vi "MyQH Main.vi"() -> ()   [LabVIEW 2014]
doc: "Diese Vorlage beschreibt das Design \"Handler für Nachrichten-Queues\".\n\nDie Schleife zur Ereignisbehandlung erzeugt Nachrichten basierend auf Benutzereingaben.\n\nDie Schleife zur Nachrichtenbehandlung verarbeitet Nachrichten, die von der Ereignisschleife oder anderen Nachrichten erzeugt wurden. Die Nachrichten sind String-Werte. Neue Nachrichten können also einfach der Case-Struktur der Nachrichtenschleife hinzugefügt werden. Der Nachrichten-Cluster kann auch einen optionalen Wert für Nachrichtendaten enthalten. Dabei handelt es sich um einen Variant, der in beliebige nachrichtenspezifische Daten umgewandelt werden kann."
uses:
  controls/ProtocolT.ctl
  controls/ProtocolEntry.ctl
  controls/MyQH UI Data.ctl
  support/Message Queue/Enqueue Message (Single).vi
  support/Message Queue/Enqueue Message (Array).vi
  <vilib>/Utility/error.llb/Error Cluster From Error Code.vi
  <vilib>/ErrorRing/Error Ring.xnode
  support/Message Queue/MyQH Message Queue.lvlib
  support/User Event - Stop/MyQH User Event - Stop.lvlib
panel:
  in  "ProtocolT":T1 {"Zeitstempel" format=" %<%X %x>T"}
  out "Anzeige <Ersetzen>":string
  in  "Remove Entry":bool
  in  "Add Entry":bool
  in  "Beenden":bool
  # "Für diese Elemente wurden Wertänderungs-Ereignisse in der Ereignisstruktur im Blockdiagramm konfiguriert.\n\nErsetzen Sie die Elemente durch für Ihre Anwendung gewünschte Elemente (und konfigurieren Sie die Ereignisstruktur neu)."
  # "Diese Vorlage beschreibt das Design für einen Handler für Nachrichten-Queues.\n\nWechseln Sie für weitere Informationen zum Blockdiagramm."
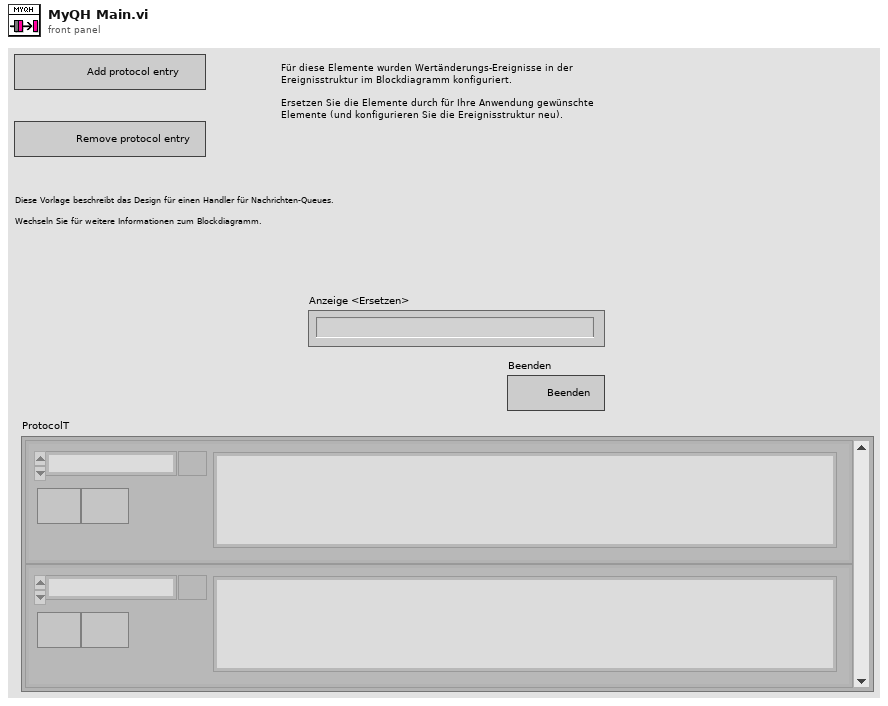
[diagram p1: front panel]
types:
  T1 = typedef "ProtocolT.ctl" = T2[]
  T2 = typedef "ProtocolEntry.ctl" = cluster{"Zeitstempel":timestamp, "String":string, "Abbrechen-Schaltfläche":bool, "Optionen-Schaltfläche":bool}
  T3 = typedef "MyQH UI Data.ctl" = cluster{"Boolesch <Ersetzen>":bool, "String <Ersetzen>":string, "Numerisch <Ersetzen>":dbl, "Etwas tun (Ref.)":refnum<vi>, "Etwas anderes tun (Ref.)":refnum<vi>, "Datenanzeige (Ref.)":refnum<vi>, "Beenden-Schaltfl. (Ref.)":refnum<vi>, "Cluster":cluster{"VI Referenz":refnum<vi>}, "Arr Referenz":refnum<vi>, "Cluster Referenz":refnum<vi>}
  T4 = cluster{"Status":bool, "Code":i32, "Quelle":string}
  T5 = typedef "MyQH Message Queue.lvlib/All Message Queues.ctl" = cluster{"UI":refnum<queue>}
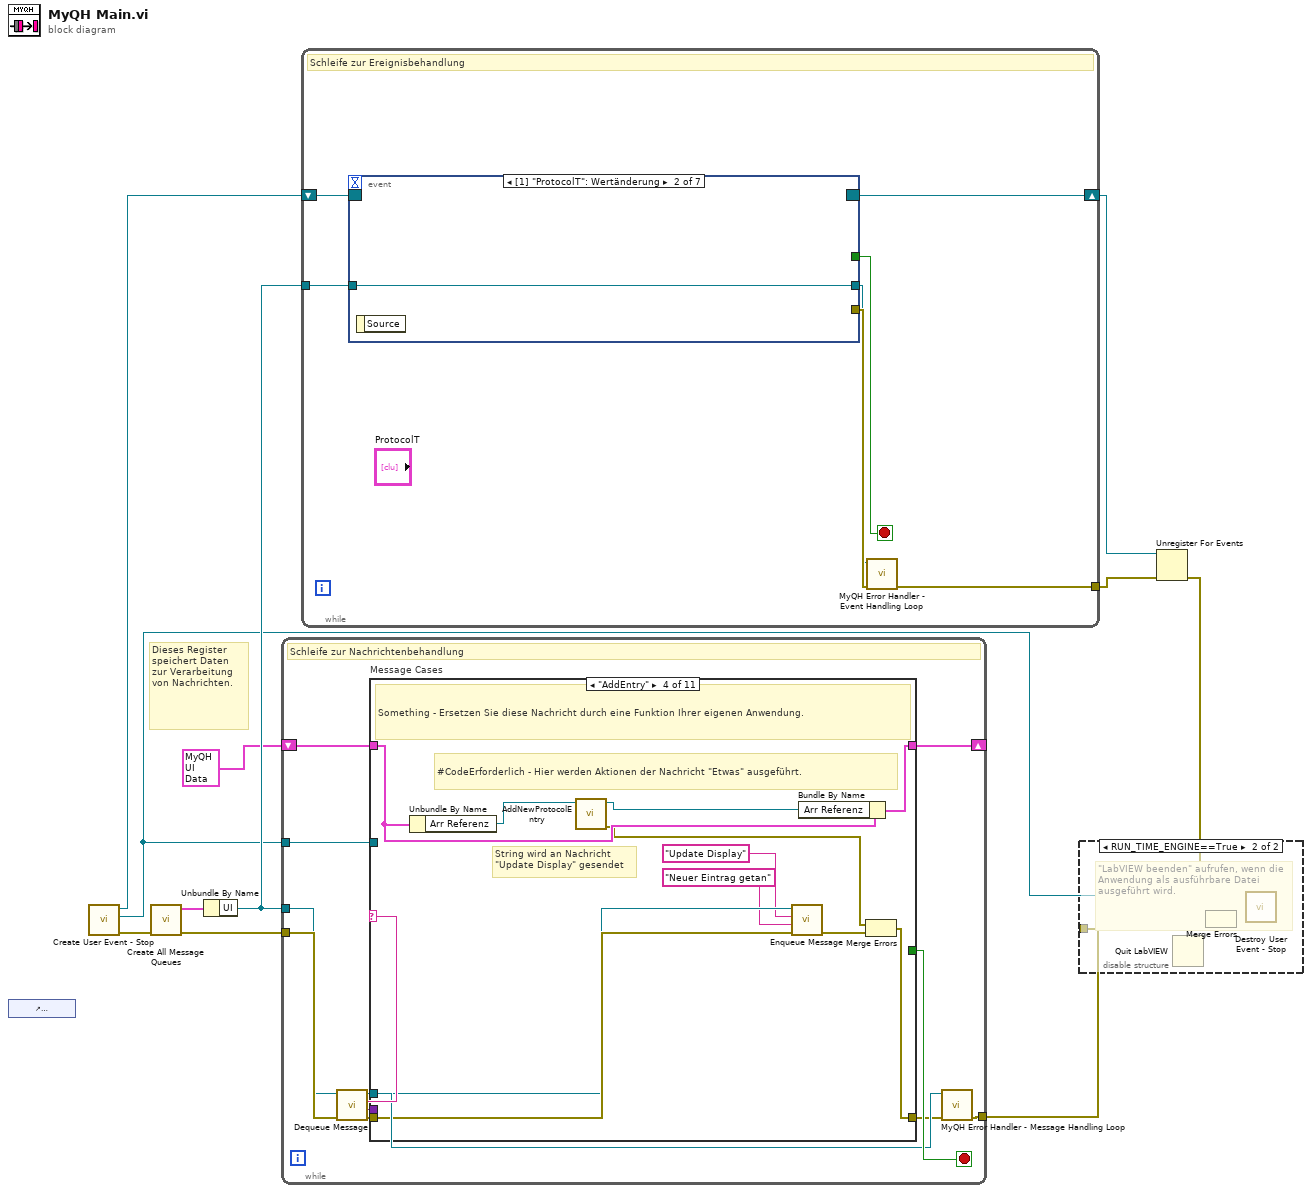
[diagram p0: block diagram]
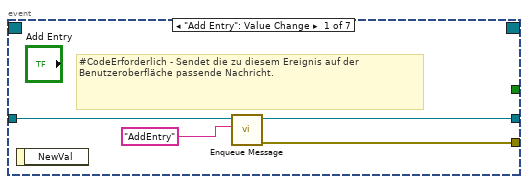
[diagram p3: hidden frame]
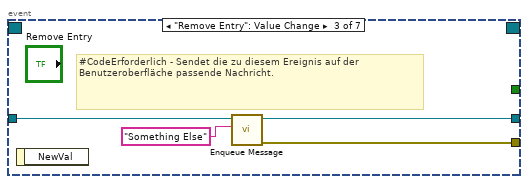
[diagram p4: hidden frame]
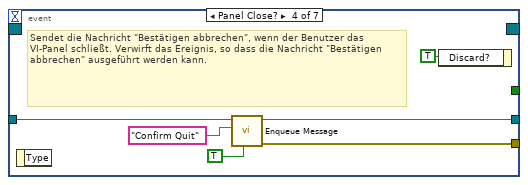
[diagram p5: hidden frame]
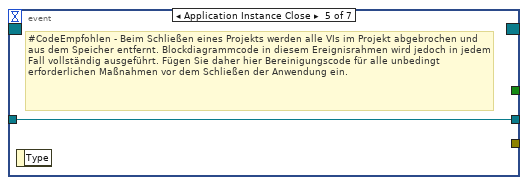
[diagram p6: hidden frame]
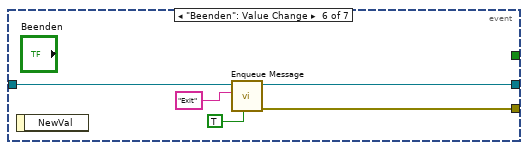
[diagram p7: hidden frame]
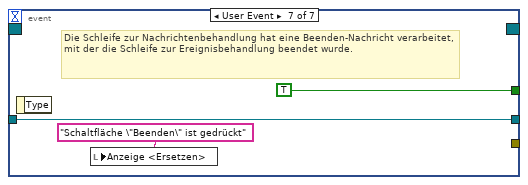
[diagram p8: hidden frame]
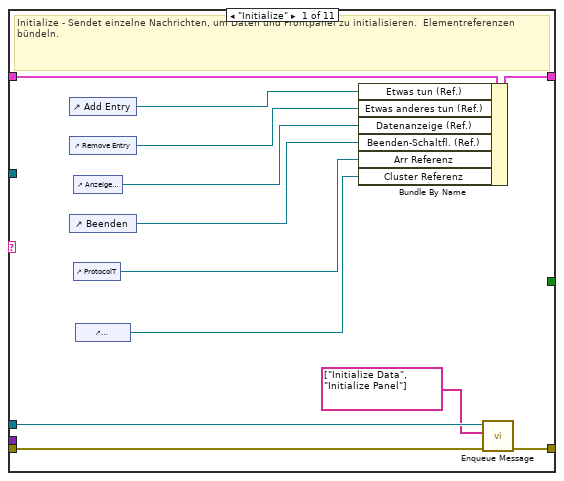
[diagram p9: hidden frame]
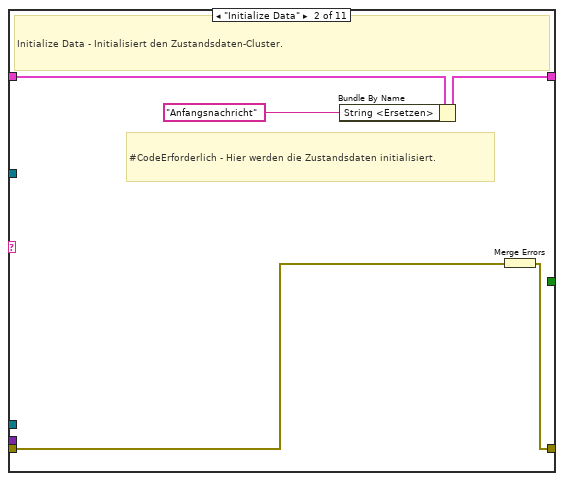
[diagram p10: hidden frame]
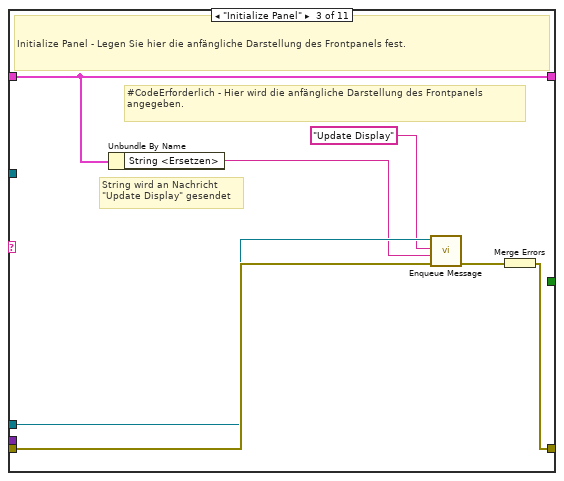
[diagram p11: hidden frame]
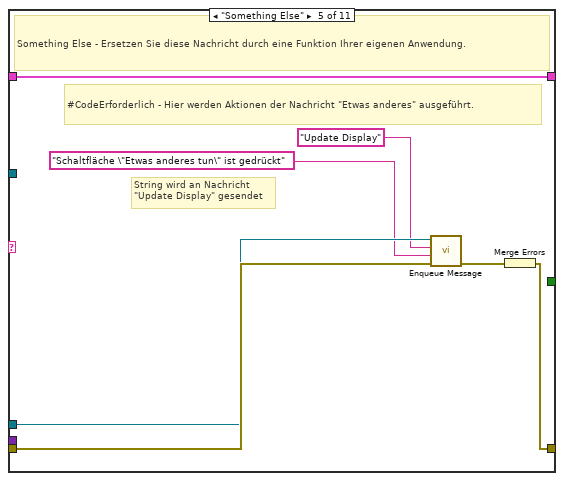
[diagram p12: hidden frame]
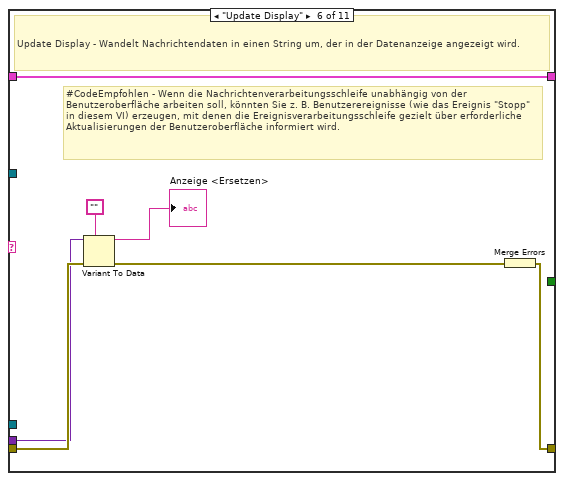
[diagram p13: hidden frame]
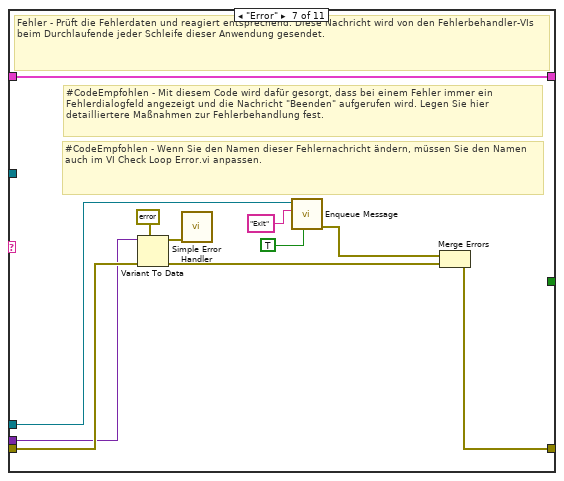
[diagram p14: hidden frame]
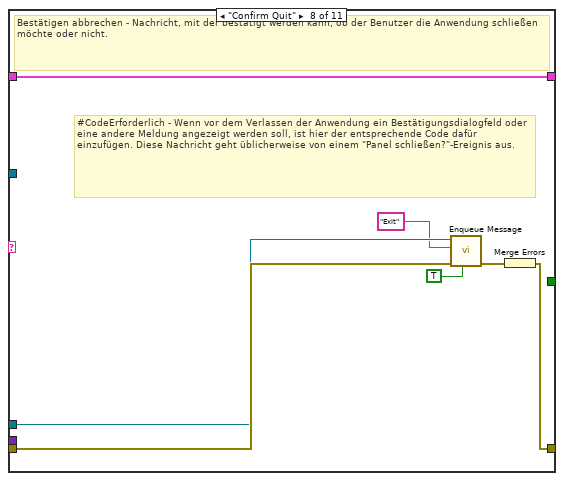
[diagram p15: hidden frame]
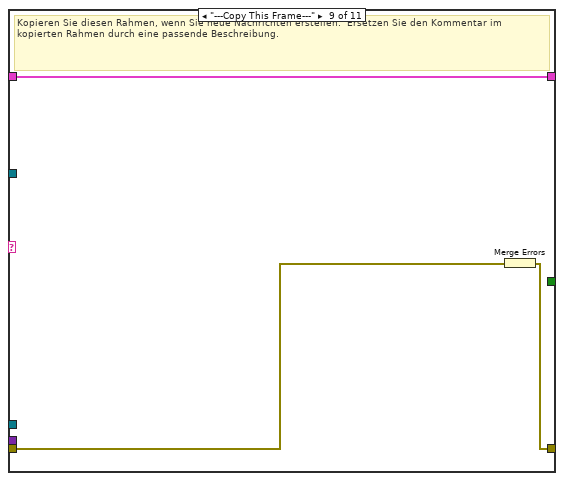
[diagram p16: hidden frame]
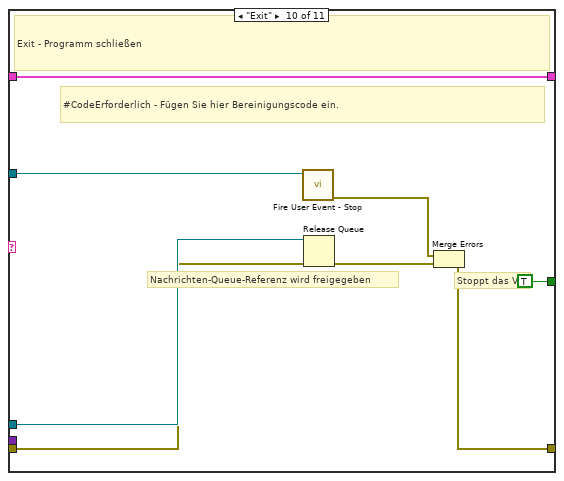
[diagram p17: hidden frame]
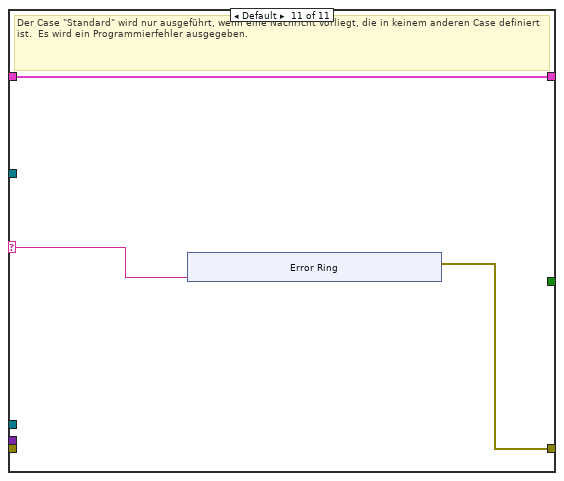
[diagram p18: hidden frame]
diagram:
  # "Dieses Register speichert Daten zur Verarbeitung von Nachrichten."
  n1 = control-ref of="Abbrechen-Schaltfläche"() -> ()  [unwired: 1 out]
  n2 = call "Create User Event - Stop.vi"() -> ("error out"=w8:T4, "Benutzerereignis - Stopp"=w6:refnum<user-event>, "Stoppereignisregistrierung (Referenz)"=w9:refnum<event-registration>)  [unwired: 9 in]
  n3 = call "Create All Message Queues.vi"("error in (no error)"=w8) -> ("error out"=w13:T4, "Nachrichten-Queues (Ausgang)"=w12:T5)  [unwired: 9 in]
  n4 = Unbundle By Name(w12) -> ("UI"=w10:refnum<queue>)
  n5 = while {
    tunnel: w10 -> [w17]
    shift-right: [w24] -> _
    shift-left: T3 {"Boolesch <Ersetzen>"=FALSE, "String <Ersetzen>"="", "Numerisch <Ersetzen>"=0.0, "Etwas tun (Ref.)"=refnum, "Etwas anderes tun (Ref.)"=refnum, "Datenanzeige (Ref.)"=refnum, "Beenden-Schaltfl. (Ref.)"=refnum, "Cluster"={"VI Referenz"=refnum}, "Arr Referenz"=refnum, "Cluster Referenz"=refnum} ("Data Cluster") -> [w25]
    tunnel: w6 -> [w22]
    tunnel: w13 -> [w21]
    tunnel: [w15] -> w11
    stop <- w23 stop-if-true
    # "Schleife zur Nachrichtenbehandlung"
    n6 = call "Dequeue Message.vi"("error in (no error)"=w21, "Nachrichten-Queue"=w17) -> ("error out"=w20:T4, "Nachrichtendaten"=w18:variant, "Nachricht"=w19:string, "Nachrichten-Queue (Kopie)"=w16:refnum<queue>)  [unwired: 6 in]
    n7 = case "Message Cases" shown="\"AddEntry\"" w19 {
      selector: w19 -> [_ _ _ _ _ _ _ _ _ _ w104]
      tunnel: w16 -> [w35 _ w46 w57 w63 _ w77 w88 _ w103 _]
      tunnel: w20 -> [w36 w42 w47 w59 w65 w72 w85 w92 w95 w98 _]
      tunnel: [w37 w38 w48 w60 w66 w73 w78 w90 w93 w99 w105] -> w14
      tunnel: w25 -> [w34 w41 w49 w52 w67 w74 w84 w91 w94 w102 w106]
      tunnel: [w33 w40 w49 w51 w67 w74 w84 w91 w94 w102 w106] -> w24
      tunnel: [_ _ _ _ _ _ _ _ _ TRUE _] -> w23
      tunnel: w18 -> [_ _ _ _ _ w71 w83 _ _ _ _]
      tunnel: w22 -> [_ _ _ _ _ _ _ _ _ w97 _]
      frame "Initialize" {
        # "Initialize - Sendet einzelne Nachrichten, um Daten und Frontpanel zu initialisieren.  Elementreferenzen bündeln."
        n8 = control-ref of="Add Entry"() -> (w32:refnum<vi>)
        n9 = control-ref of="Remove Entry"() -> (w31:refnum<vi>)
        n10 = control-ref of="Beenden"() -> (w29:refnum<vi>)
        n11 = control-ref of="Anzeige <Ersetzen>"() -> (w30:refnum<vi>)
        n12 = control-ref of="ProtocolT"() -> (w27:refnum<vi>)
        n13 = control-ref of="ProtocolEntryT"() -> (w26:refnum<vi>)
        n14 = Bundle By Name(cluster=w34, "Etwas tun (Ref.)"=w32, "Etwas anderes tun (Ref.)"=w31, "Datenanzeige (Ref.)"=w30, "Beenden-Schaltfl. (Ref.)"=w29, "Arr Referenz"=w27, "Cluster Referenz"=w26) -> (w33:T3)
        n15 = call-poly "Enqueue Message.vi"("error in (no error)"=w36, "Nachrichten-Array"=string[] ["Initialize Data", "Initialize Panel"], "Nachrichten-Queue"=w35) -> ("error out"=w37:T4)  [unwired: 7 in, 1 out]
      }
      frame "Initialize Data" {
        # "#CodeErforderlich - Hier werden die Zustandsdaten initialisiert."
        # "Initialize Data - Initialisiert den Zustandsdaten-Cluster."
        n16 = Bundle By Name(cluster=w41, "String <Ersetzen>"="Anfangsnachricht" ("Initial Message")) -> (w40:T3)
        n17 = Merge Errors(w42) -> (w38:errorcluster)
      }
      frame "Initialize Panel" {
        # "String wird an Nachricht\n\"Update Display\" gesendet"
        # "#CodeErforderlich - Hier wird die anfängliche Darstellung des Frontpanels angegeben."
        # "Initialize Panel - Legen Sie hier die anfängliche Darstellung des Frontpanels fest."
        n18 = Unbundle By Name(w49) -> ("String <Ersetzen>"=w43:string)
        n19 = call-poly "Enqueue Message.vi"("error in (no error)"=w47, "Nachrichtendaten"=w43, "Nachricht"="Update Display" ("Message"), "Nachrichten-Queue"=w46) -> ("error out"=w45:T4)  [unwired: 6 in, 1 out]
        n20 = Merge Errors(w45) -> (w48:errorcluster)
      }
      frame "AddEntry" {
        # "String wird an Nachricht\n\"Update Display\" gesendet"
        # "#CodeErforderlich - Hier werden Aktionen der Nachricht \"Etwas\" ausgeführt."
        # "Something - Ersetzen Sie diese Nachricht durch eine Funktion Ihrer eigenen Anwendung."
        n21 = Unbundle By Name(w52) -> ("Arr Referenz"=w54:refnum<vi>)
        n22 = call "AddNewProtocolEntry.vi"("Array (Eingang)"=w54) -> ("Fehler (Ausgang)"=w50:errorcluster, "Referenz (Ausgang)"=w53:refnum<vi>)  [unwired: 9 in]
        n23 = call-poly "Enqueue Message.vi"("error in (no error)"=w59, "Nachrichtendaten"="Neuer Eintrag getan" ("\"Do Something\" button pressed"), "Nachricht"="Update Display" ("Message"), "Nachrichten-Queue"=w57) -> ("error out"=w58:T4)  [unwired: 6 in, 1 out]
        n24 = Bundle By Name(cluster=w52, "Arr Referenz"=w53) -> (w51:T3)
        n25 = Merge Errors(w50, w58) -> (w60:errorcluster)
      }
      frame "Something Else" {
        # "String wird an Nachricht\n\"Update Display\" gesendet"
        # "#CodeErforderlich - Hier werden Aktionen der Nachricht \"Etwas anderes\" ausgeführt."
        # "Something Else - Ersetzen Sie diese Nachricht durch eine Funktion Ihrer eigenen Anwendung."
        n26 = call-poly "Enqueue Message.vi"("error in (no error)"=w65, "Nachrichtendaten"="Schaltfläche \"Etwas anderes tun\" ist gedrückt" ("\"Do Something Else\" button pressed"), "Nachricht"="Update Display" ("Message"), "Nachrichten-Queue"=w63) -> ("error out"=w64:T4)  [unwired: 6 in, 1 out]
        n27 = Merge Errors(w64) -> (w66:errorcluster)
      }
      frame "Update Display" {
        # "#CodeEmpfohlen - Wenn die Nachrichtenverarbeitungsschleife unabhängig von der Benutzeroberfläche arbeiten soll, könnten Sie z. B. Benutzerereignisse (wie das Ereignis \"Stopp\" in diesem VI) erzeugen, mit denen die Ereignisverarbeitungsschleife gezielt über erforderliche Aktualisierungen der Benutzeroberfläche informiert wird."
        # "Update Display - Wandelt Nachrichtendaten in einen String um, der in der Datenanzeige angezeigt wird."
        n28 = Variant To Data(error in=w72, type="", Variant=w71) -> (data=→"Anzeige <Ersetzen>":string, error out=w69:errorcluster)
        n29 = Merge Errors(w69) -> (w73:errorcluster)
      }
      frame "Error" {
        # "#CodeEmpfohlen - Wenn Sie den Namen dieser Fehlernachricht ändern, müssen Sie den Namen auch im VI Check Loop Error.vi anpassen."
        # "#CodeEmpfohlen - Mit diesem Code wird dafür gesorgt, dass bei einem Fehler immer ein Fehlerdialogfeld angezeigt und die Nachricht \"Beenden\" aufgerufen wird. Legen Sie hier detailliertere Maßnahmen zur Fehlerbehandlung fest."
        # "Fehler - Prüft die Fehlerdaten und reagiert entsprechend. Diese Nachricht wird von den Fehlerbehandler-VIs beim Durchlaufende jeder Schleife dieser Anwendung gesendet."
        n30 = Variant To Data(error in=w85, type=errorcluster {"status"=FALSE, "code"=0, "source"=""} ("error constant"), Variant=w83) -> (data=w81:errorcluster, error out=w80:errorcluster)
        n31 = call <vilib>:"Simple Error Handler.vi"("error in (no error)"=w81) -> ()  [unwired: 4 in, 5 out]
        n32 = call-poly "Enqueue Message.vi"("Nachricht mit Priorität? (F)"=TRUE ("Priority Message? (F)"), "Nachricht"="Exit", "Nachrichten-Queue"=w77) -> ("error out"=w79:T4)  [unwired: 7 in, 1 out]
        n33 = Merge Errors(w79, w80) -> (w78:errorcluster)
      }
      frame "Confirm Quit" {
        # "#CodeErforderlich - Wenn vor dem Verlassen der Anwendung ein Bestätigungsdialogfeld oder eine andere Meldung angezeigt werden soll, ist hier der entsprechende Code dafür einzufügen. Diese Nachricht geht üblicherweise von einem \"Panel schließen?\"-Ereignis aus."
        # "Bestätigen abbrechen - Nachricht, mit der bestätigt werden kann, ob der Benutzer die Anwendung schließen möchte oder nicht."
        n34 = call-poly "Enqueue Message.vi"("Nachricht mit Priorität? (F)"=TRUE ("Priority Message? (F)"), "error in (no error)"=w92, "Nachricht"="Exit" ("Message"), "Nachrichten-Queue"=w88) -> ("error out"=w89:T4)  [unwired: 6 in, 1 out]
        n35 = Merge Errors(w89) -> (w90:errorcluster)
      }
      frame "---Copy This Frame---" {
        # "Kopieren Sie diesen Rahmen, wenn Sie neue Nachrichten erstellen.  Ersetzen Sie den Kommentar im kopierten Rahmen durch eine passende Beschreibung."
        n36 = Merge Errors(w95) -> (w93:errorcluster)
      }
      frame "Exit" {
        # "Stoppt das VI."
        # "Nachrichten-Queue-Referenz wird freigegeben"
        # "#CodeErforderlich - Fügen Sie hier Bereinigungscode ein."
        # "Exit - Programm schließen"
        n37 = call "Fire User Event - Stop.vi"("Benutzerereignis - Stopp"=w97) -> ("error out"=w96:T4)  [unwired: 10 in]
        n38 = Release Queue(queue=w103, error in (no error)=w98) -> (error out=w100:errorcluster)  [unwired: 1 in, 2 out]
        n39 = Merge Errors(w96, w100) -> (w99:errorcluster)
      }
      frame Default {
        # "Der Case \"Standard\" wird nur ausgeführt, wenn eine Nachricht vorliegt, die in keinem anderen Case definiert ist.  Es wird ein Programmierfehler ausgegeben."
        n40 = xnode "Error Ring"("Parameter 0"=w104) -> ("Fehler (Ausgang)"=w105:errorcluster)
      }
    }
    n41 = call "MyQH Error Handler - Message Handling Loop.vi"("error in (no error)"=w14, "Nachrichten-Queue"=w16) -> ("Fehler (Eingang, Kopie)"=w15:T4)  [unwired: 8 in, 1 out]
  }
  n42 = while {
    tunnel: w10 -> [w120]
    shift-right: [w118] -> w4
    shift-left: w9 -> [w119]
    tunnel: [w114] -> w1
    stop <- w116 stop-if-true
    # "Schleife zur Ereignisbehandlung"
    n43 = event shown="[1] \"ProtocolT\": Wertänderung" {
      selector: w119 -> [_ _ _ _ _ _ _]
      dyn-events: [_ _ _ _ _ _ _] -> w118
      timeout: _ -> [_ _ _ _ _ _ _]
      tunnel: [_ _ _ _ _ _ TRUE ("Discard?")] -> w116
      tunnel: w120 -> [w124 w125 w129 w134 w136 w141 w144]
      tunnel: [w121 _ w126 w133 _ w140 _] -> w117
      tunnel: [w123 w125 w128 w132 w136 w139 w144] -> w115
      event "Add Entry": Value Change {
        # "#CodeErforderlich - Sendet die zu diesem Ereignis auf der Benutzeroberfläche passende Nachricht."
        n44 = event-data() -> ()  [unwired: 1 in, 1 out]
        n45 = call-poly "Enqueue Message.vi"("Nachricht"="AddEntry" ("Message"), "Nachrichten-Queue"=w124) -> ("error out"=w121:T4, "Nachrichten-Queue (Kopie)"=w123:refnum<queue>)  [unwired: 8 in]
      }
      event Value Change {
        n46 = event-data() -> ()  [unwired: 1 in, 1 out]
      }
      event "Remove Entry": Value Change {
        # "#CodeErforderlich - Sendet die zu diesem Ereignis auf der Benutzeroberfläche passende Nachricht."
        n47 = event-data() -> ()  [unwired: 1 in, 1 out]
        n48 = call-poly "Enqueue Message.vi"("Nachricht"="Something Else" ("Message"), "Nachrichten-Queue"=w129) -> ("error out"=w126:T4, "Nachrichten-Queue (Kopie)"=w128:refnum<queue>)  [unwired: 8 in]
      }
      event Panel Close? {
        # "Sendet die Nachricht \"Bestätigen abbrechen\", wenn der Benutzer das VI-Panel schließt. Verwirft das Ereignis, so dass die Nachricht \"Bestätigen abbrechen\" ausgeführt werden kann."
        n49 = event-data() -> ()  [unwired: 1 in, 1 out]
        n50 = call-poly "Enqueue Message.vi"("Nachricht mit Priorität? (F)"=TRUE ("Priority Message? (F)"), "Nachricht"="Confirm Quit" ("Message"), "Nachrichten-Queue"=w134) -> ("error out"=w133:T4, "Nachrichten-Queue (Kopie)"=w132:refnum<queue>)  [unwired: 7 in]
        n51 = event-data("Discard?"=TRUE) -> ()  [unwired: 1 in, 1 out]
      }
      event Application Instance Close {
        # "#CodeEmpfohlen - Beim Schließen eines Projekts werden alle VIs im Projekt abgebrochen und aus dem Speicher entfernt. Blockdiagrammcode in diesem Ereignisrahmen wird jedoch in jedem Fall vollständig ausgeführt. Fügen Sie daher hier Bereinigungscode für alle unbedingt erforderlichen Maßnahmen vor dem Schließen der Anwendung ein."
        n52 = event-data() -> ()  [unwired: 1 in, 1 out]
      }
      event "Beenden": Value Change {
        n53 = event-data() -> ()  [unwired: 1 in, 1 out]
        n54 = call-poly "Enqueue Message.vi"("Nachricht mit Priorität? (F)"=TRUE ("Priority Message? (F)"), "Nachricht"="Exit" ("Message"), "Nachrichten-Queue"=w141) -> ("error out"=w140:T4, "Nachrichten-Queue (Kopie)"=w139:refnum<queue>)  [unwired: 7 in]
      }
      event User Event {
        # "Die Schleife zur Nachrichtenbehandlung hat eine Beenden-Nachricht verarbeitet, mit der die Schleife zur Ereignisbehandlung beendet wurde."
        n55 = event-data() -> ()  [unwired: 1 in, 1 out]
        n56 = local write "Anzeige <Ersetzen>"("Schaltfläche \"Beenden\" ist gedrückt" ("VI Stopped")) -> ()
      }
    }
    n57 = call "MyQH Error Handler - Event Handling Loop.vi"("error in (no error)"=w117, "Nachrichten-Queue"=w115) -> ("Fehler (Eingang, Kopie)"=w114:T4)  [unwired: 8 in, 1 out]
  }
  n58 = Unregister For Events(event registration refnum=w4, error in=w1) -> (error out=w5:errorcluster)
  n59 = Merge Errors(w5, w11) -> (w7:errorcluster)
  n60 = call "Destroy User Event - Stop.vi"("error in (no error)"=w7, "Benutzerereignis - Stopp"=w6) -> ("error out"=w2:T4)  [unwired: 9 in]
  n61 = disable-structure shown="RUN_TIME_ENGINE==True" {
    disable-tunnel: w2 -> [_ _]
    frame condition #0 (active) {
    }
    frame condition #1 {
      # "\"LabVIEW beenden\" aufrufen, wenn die Anwendung als ausführbare Datei ausgeführt wird."
      n62 = Quit LabVIEW() -> ()  [unwired: 1 in]
    }
  }
